vi "ModifyChannelInfo.vi"(9 "新通道信息":T1, 10 "通道索引":i32, 11 "原通道名称":string) -> ()   [LabVIEW 2018, in "DataDisplay.lvlib"]
uses:
  DataDisplay.lvlib
  TypeDefine/DD_ChannelInfo.ctl
  DD_Parameter.vi
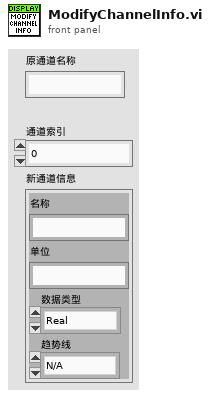
[diagram p1: front panel]
types:
  T1 = typedef "DataDisplay.lvlib/DD_ChannelInfo.ctl" = cluster{"名称":string, "单位":string, "数据类型":enum16{"Real", "Int"}, "趋势线":enum16{"N/A", "X", "Y"}}
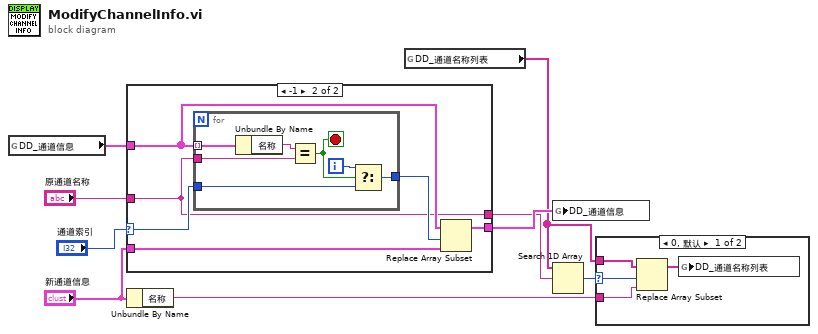
[diagram p0: block diagram]
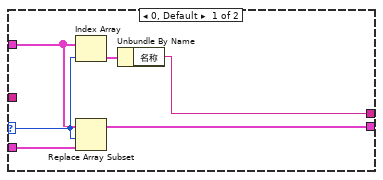
[diagram p3: hidden frame]
diagram:
  n1 = global read "DD_Parameter.vi" "DD_通道信息"() -> (w8:T1[])
  n2 = case shown="-1" "通道索引" {
    selector: "通道索引" -> [w13 w21]
    tunnel: w8 -> [w12 w20]
    tunnel: [w14 w16] -> w5
    tunnel: "原通道名称" -> [_ w16]
    tunnel: "新通道信息" -> [w11 w18]
    tunnel: [w10 w17] -> w6
    frame 0, Default {
      n3 = Index Array(array=w12, index=w13) -> (element=w15:T1)
      n4 = Replace Array Subset(array=w12, new element=w11, index=w13) -> (w10:T1[])
      n5 = Unbundle By Name(w15) -> ("名称"=w14:string)
    }
    frame -1 {
      n6 = for {
        tunnel: w20 -> [w28] mode=indexing
        tunnel: w16 -> [w27]
        tunnel: w21 -> [w23]
        tunnel: [w22] -> w19
        i -> [w24]
        stop <- w25 stop-if-true
        n7 = Unbundle By Name(w28) -> ("名称"=w26:string)
        n8 = Equal?(x=w26, y=w27) -> (x = y?=w25:bool)
        n9 = Select(t=w24, s=w25, f=w23) -> (s? t:f=w22:i32)
      }
      n10 = Replace Array Subset(array=w20, new element=w18, index=w19) -> (w17:T1[])
    }
  }
  n11 = Unbundle By Name("新通道信息") -> ("名称"=w2:string)
  n12 = global read "DD_Parameter.vi" "DD_通道名称列表"() -> (w1:string[])
  n13 = global write "DD_Parameter.vi" "DD_通道信息"(w6) -> ()
  n14 = Search 1D Array(1D array=w1, element=w5) -> (index of element=w4:i32)  [unwired: 1 in]
  n15 = case shown="0, 默认" w4 {
    selector: w4 -> [w32 _]
    tunnel: w2 -> [w31 _]
    tunnel: w1 -> [w30 _]
    frame 0, Default {
      n16 = Replace Array Subset(array=w30, new element=w31, index=w32) -> (w29:string[])
      n17 = global write "DD_Parameter.vi" "DD_通道名称列表"(w29) -> ()
    }
    frame -1 {
    }
  }
